vi "raspberry_producemt_consumer.vi"() -> ()   [LabVIEW 2020]
uses:
  Cmd_enum.ctl
  Parameters_cluster.ctl
  ToConsumentData_cluster.ctl
  BaudRate_enum.ctl
  <vilib>/Instr/_visa.llb/VISA Configure Serial Port (Instr).vi
panel:
  in  "Baud Rate":enum32{"9600", "115200"}(ring)
  in  "Serial Port":refnum<visa-resource-name>="N/A"
  out "Logs":string
  out "Chart":dbl(graph)
  in  "Stop":bool
  in  "Disconnect":bool
  in  "Connect":bool
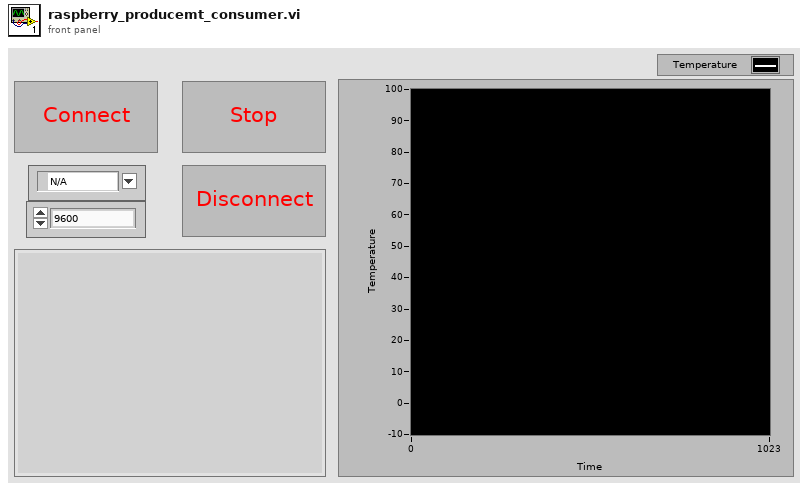
[diagram p1: front panel]
types:
  T1 = typedef "ToConsumentData_cluster.ctl" = cluster{"Cmd":T2, "Param":T3}
  T2 = typedef "Cmd_enum.ctl" = enum16{"Init", "Connect", "Disconnect", "ReadData", "Exit"}
  T3 = typedef "Parameters_cluster.ctl" = cluster{"Stop":bool, "Connect":bool, "Disconnect":bool, "Port COM":refnum<visa-resource-name>, "Enum":T4}
  T4 = typedef "BaudRate_enum.ctl" = enum16{"115200", "9600"}
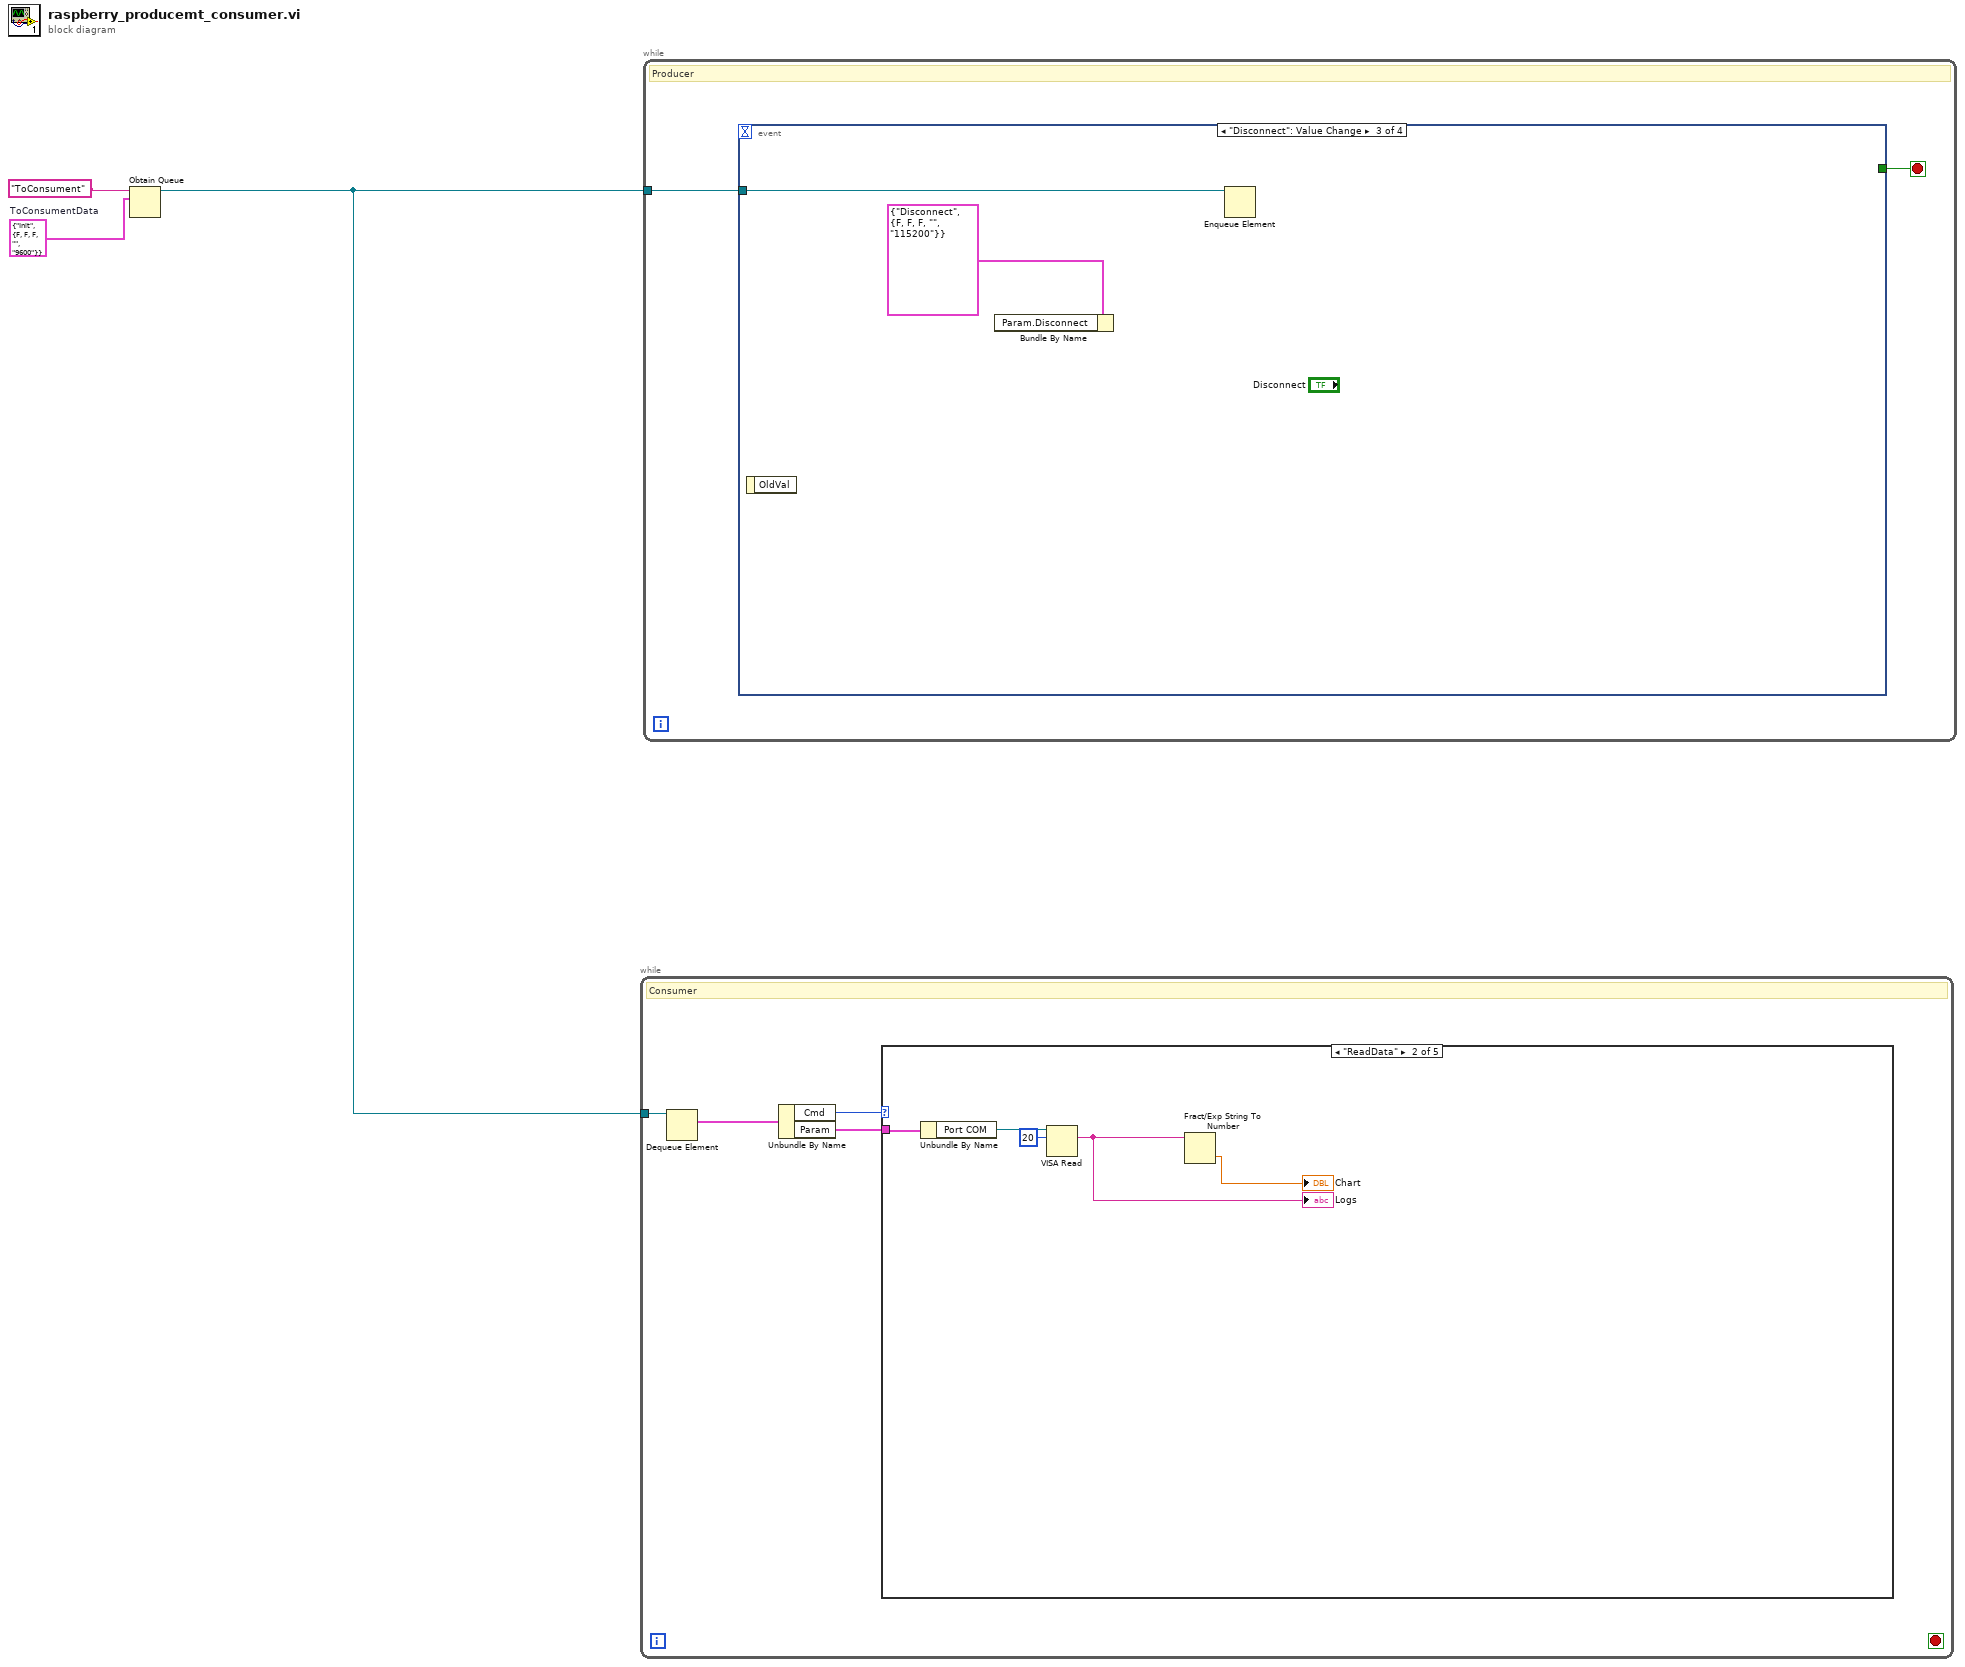
[diagram p0: block diagram]
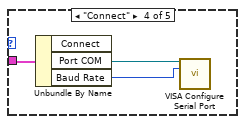
[diagram p4: hidden frame]
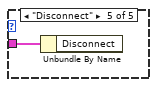
[diagram p5: hidden frame]
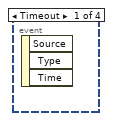
[diagram p6: hidden frame]
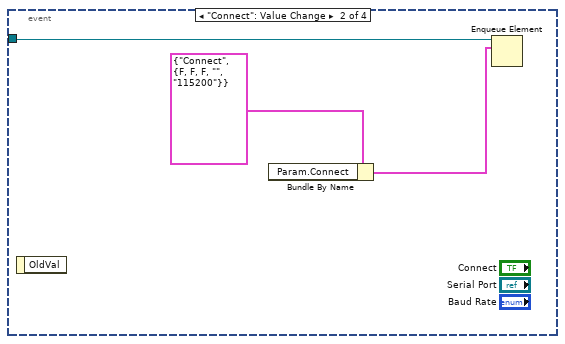
[diagram p7: hidden frame]
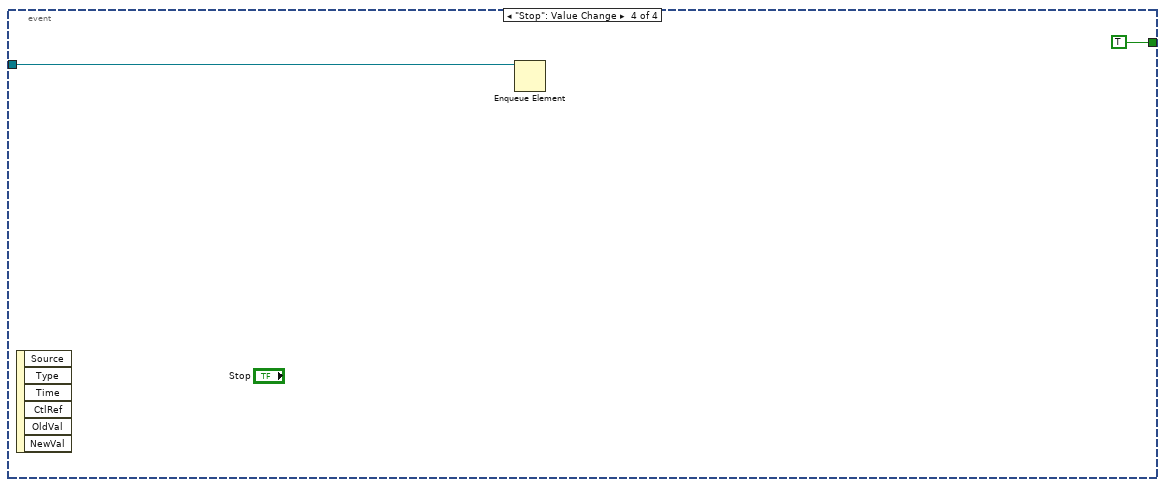
[diagram p8: hidden frame]
diagram:
  w1 = T1 {"Cmd"=enum."Init", "Param"={"Stop"=FALSE, "Connect"=FALSE, "Disconnect"=FALSE, "Port COM"="", "Enum"=enum."9600"}}  # ToConsumentData
  n1 = Obtain Queue(name (unnamed)="ToConsument", element data type=w1) -> (queue out=w2:refnum<queue>)  [unwired: 3 in, 2 out]
  n2 = while {
    tunnel: w2 -> [w7]
    stop <- _ stop-if-true
    # "Consumer"
    n3 = Dequeue Element(queue=w7) -> (element=w6:T1)  [unwired: 2 in, 3 out]
    n4 = Unbundle By Name(w6) -> ("Cmd"=w5:T2, "Param"=w4:T3)
    n5 = case shown="\"ReadData\"" w5 {
      tunnel: w4 -> [_ w12 _ w15 w16]
      frame "Init", Default {
      }
      frame "ReadData" {
        n6 = Unbundle By Name(w12) -> ("Port COM"=w11:refnum<visa-resource-name>)
        n7 = VISA Read(VISA resource name=w11, byte count=u32 20) -> (read buffer=w10:string)  [unwired: 1 in, 3 out]
        "Logs" <- w10
        n8 = Fract/Exp String To Number(string=w10) -> (number=→"Chart":dbl)  [unwired: 3 in, 1 out]
      }
      frame "Exit" {
      }
      frame "Connect" {
        n9 = Unbundle By Name(w15) -> ("Port COM"=w14:refnum<visa-resource-name>, "Baud Rate"=w13:u32)  [unwired: 1 out]
        n10 = call-poly "VISA Configure Serial Port"("VISA resource name"=w14, "baud rate (9600)"=w13) -> ()  [unwired: 12 in, 2 out]
      }
      frame "Disconnect" {
        n11 = Unbundle By Name(w16) -> ()  [unwired: 1 out]
      }
    }
  }
  n12 = while {
    tunnel: w2 -> [w18]
    stop <- w17 stop-if-true
    # "Producer"
    n13 = event shown="[2] \"Disconnect\": Value Change" {
      selector: _ -> [_ _ _ _]
      dyn-events: _ -> [_ _ _ _]
      timeout: _ -> [_ _ _ _]
      tunnel: w18 -> [_ w21 w23 w25]
      tunnel: [_ _ _ TRUE] -> w17
      event Timeout {
        n14 = event-data() -> ()  [unwired: 1 in, 3 out]
      }
      event "Connect": Value Change {
        n15 = event-data() -> ()  [unwired: 1 in, 1 out]
        n16 = Bundle By Name(cluster=T1 {"Cmd"=enum."Connect", "Param"={"Stop"=FALSE, "Connect"=FALSE, "Disconnect"=FALSE, "Port COM"="", "Enum"=enum."115200"}} ("element")) -> (w19:T1)  [unwired: 1 in]
        n17 = Enqueue Element(queue=w21, element=w19) -> ()  [unwired: 2 in, 3 out]
      }
      event "Disconnect": Value Change {
        n18 = event-data() -> ()  [unwired: 1 in, 1 out]
        n19 = Bundle By Name(cluster=T1 {"Cmd"=enum."Disconnect", "Param"={"Stop"=FALSE, "Connect"=FALSE, "Disconnect"=FALSE, "Port COM"="", "Enum"=enum."115200"}} ("element")) -> ()  [unwired: 1 in, 1 out]
        n20 = Enqueue Element(queue=w23) -> ()  [unwired: 3 in, 3 out]
      }
      event "Stop": Value Change {
        n21 = event-data() -> ()  [unwired: 1 in, 6 out]
        n22 = Enqueue Element(queue=w25) -> ()  [unwired: 3 in, 3 out]
      }
    }
  }
